vi "CoinInsert.vi"(3 "Error In":errorcluster) -> (0 "Error Out":errorcluster, 1 "wrzucona kwota":string, 2 "Numeric":dbl format="%.2g")   [LabVIEW 2023]
uses:
  ctls/10gr.ctl
  ctls/20gr.ctl
  ctls/50gr.ctl
  ctls/1zloty.ctl
  ctls/2zlote.ctl
  ctls/5zlotych.ctl
panel:
  in  "zakończ":T1
  in  "5zł":T2
  in  "2zł":T3
  in  "1zł":T4
  in  "50gr":T5
  in  "20gr":T6
  in  "10gr":T1
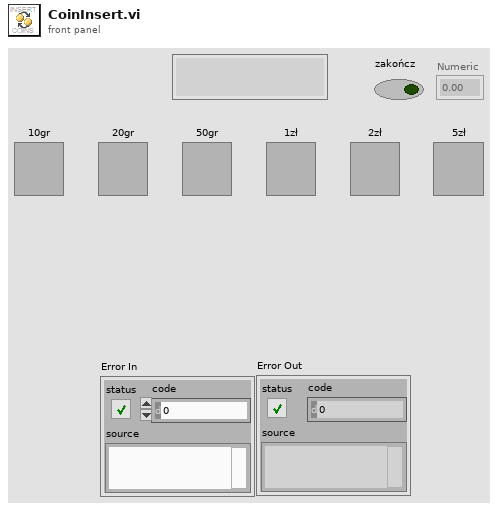
[diagram p1: front panel]
types:
  T1 = typedef "10gr.ctl" = bool
  T2 = typedef "5zlotych.ctl" = bool
  T3 = typedef "2zlote.ctl" = bool
  T4 = typedef "1zloty.ctl" = bool
  T5 = typedef "50gr.ctl" = bool
  T6 = typedef "20gr.ctl" = bool
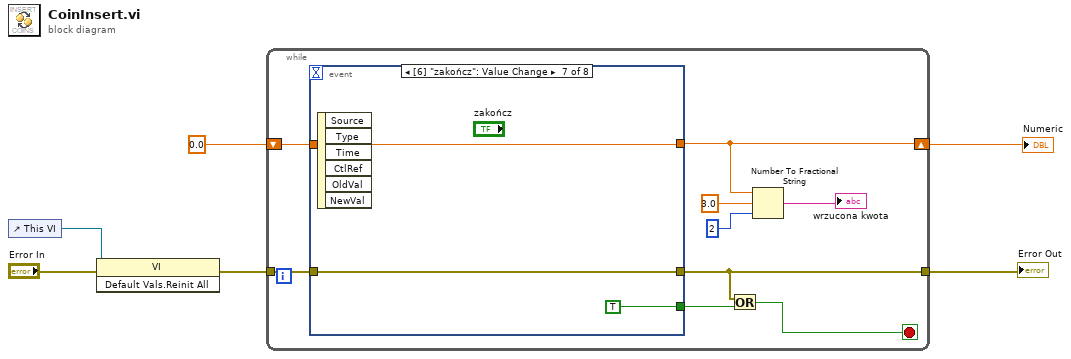
[diagram p0: block diagram]
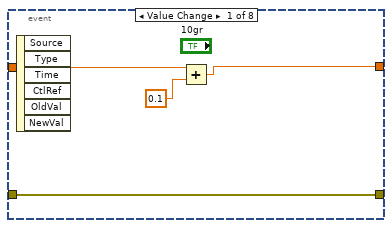
[diagram p2: hidden frame]
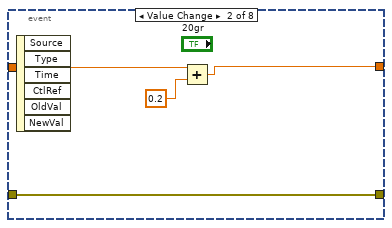
[diagram p3: hidden frame]
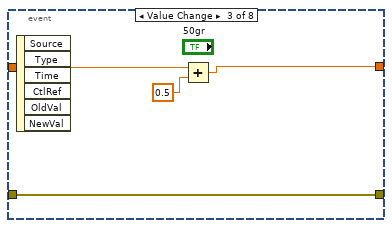
[diagram p4: hidden frame]
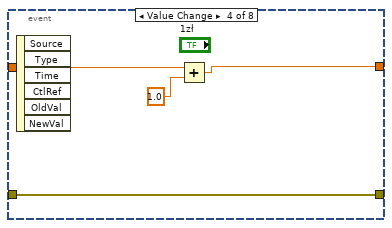
[diagram p5: hidden frame]
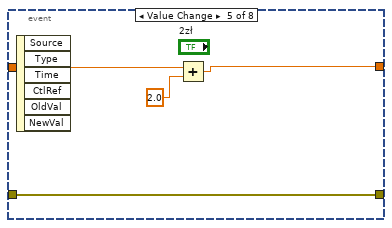
[diagram p6: hidden frame]
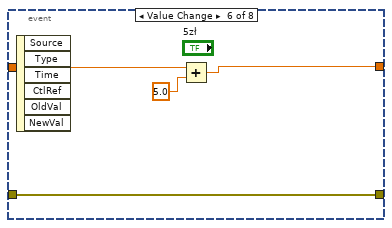
[diagram p7: hidden frame]
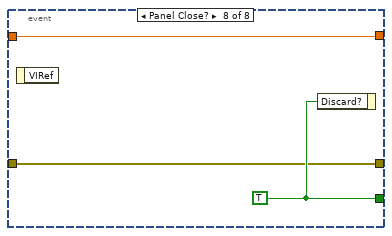
[diagram p8: hidden frame]
diagram:
  n1 = control-ref of="This VI"() -> (w5:refnum<vi>)
  n2 = invoke class="VI" method="Default Vals.Reinit All"(reference=w5, error in="Error In") -> (error out=w4:errorcluster)  [unwired: 1 in, 2 out]
  n3 = while {
    tunnel: w4 -> [w15]
    tunnel: [w13] -> w3
    shift-right: [w10] -> w1
    shift-left: 0.0 -> [w12]
    stop <- w14 stop-if-true
    n4 = event shown="[6] \"zakończ\": Value Change" {
      selector: _ -> [_ _ _ _ _ _ _ _]
      dyn-events: _ -> [_ _ _ _ _ _ _ _]
      timeout: _ -> [_ _ _ _ _ _ _ _]
      tunnel: [w16 w20 w24 w28 w32 w38 w40 w43] -> w13
      tunnel: w15 -> [w16 w20 w24 w28 w32 w38 w40 w43]
      tunnel: w12 -> [w18 w21 w25 w30 w33 w37 w42 w44]
      tunnel: [w19 w22 w26 w29 w34 w36 w42 w44] -> w10
      tunnel: [_ _ _ _ _ _ TRUE w45] -> w11
      event Value Change {
        n5 = event-data() -> ()  [unwired: 1 in, 6 out]
        n6 = Add(x=w18, y=0.1) -> (x+y=w19:dbl)
      }
      event Value Change {
        n7 = event-data() -> ()  [unwired: 1 in, 6 out]
        n8 = Add(x=w21, y=0.2) -> (x+y=w22:dbl)
      }
      event Value Change {
        n9 = event-data() -> ()  [unwired: 1 in, 6 out]
        n10 = Add(x=w25, y=0.5) -> (x+y=w26:dbl)
      }
      event Value Change {
        n11 = event-data() -> ()  [unwired: 1 in, 6 out]
        n12 = Add(x=w30, y=1.0) -> (x+y=w29:dbl)
      }
      event Value Change {
        n13 = event-data() -> ()  [unwired: 1 in, 6 out]
        n14 = Add(x=w33, y=2.0) -> (x+y=w34:dbl)
      }
      event Value Change {
        n15 = event-data() -> ()  [unwired: 1 in, 6 out]
        n16 = Add(x=w37, y=5.0) -> (x+y=w36:dbl)
      }
      event Value Change {
        n17 = event-data() -> ()  [unwired: 1 in, 6 out]
      }
      event Panel Close? {
        w45 = TRUE
        n18 = event-data() -> ()  [unwired: 1 in, 1 out]
        n19 = event-data("Discard?"=w45) -> ()  [unwired: 1 in, 1 out]
      }
    }
    n20 = Or(x=w13, y=w11) -> (x .or. y?=w14:bool)
    n21 = Number To Fractional String(number=w10, width (-)=3.0, precision (6)=i16 2) -> (F-format string=→"wrzucona kwota":string)  [unwired: 1 in]
  }
  "Error Out" <- w3
  "Numeric" <- w1
